vi "Snooze(SubVI).vi"(10 "snooze":dbl, 11 "Time hh::mm":string) -> (3 "Time hh::mm + snooze":string)   [LabVIEW 2023]
doc: "Adds snooze to input time"
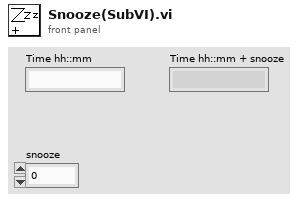
[diagram p1: front panel]
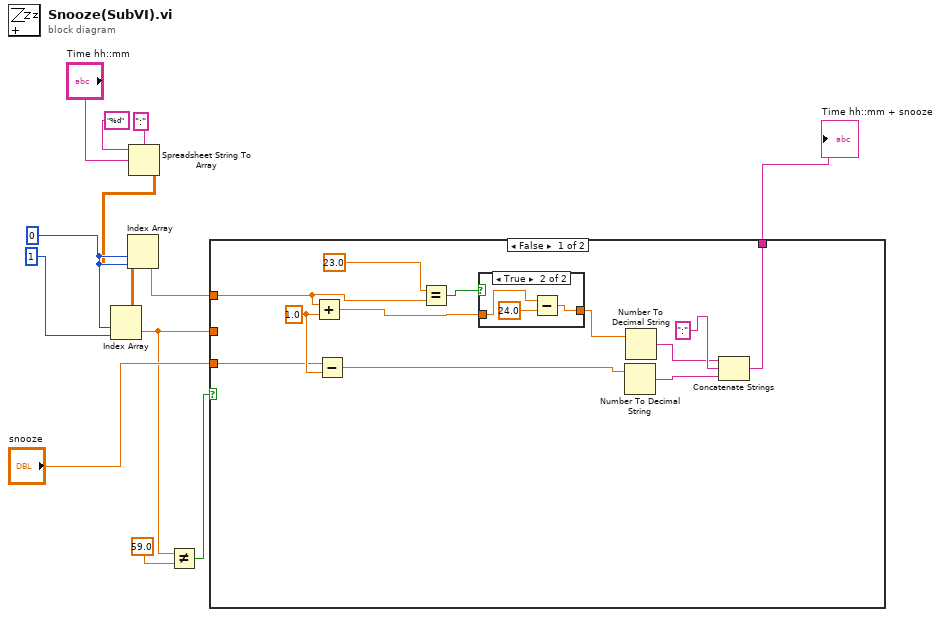
[diagram p0: block diagram]
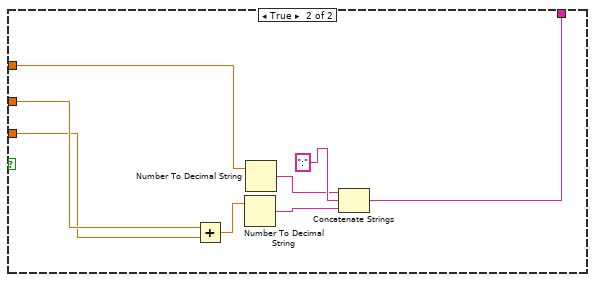
[diagram p3: hidden frame]
diagram:
  w12 = 0 ("index (row)")
  n1 = Spreadsheet String To Array(delimiter (Tab)=":", format string="%d", spreadsheet string="Time hh::mm") -> (array=w8:dbl[][])  [unwired: 1 in]
  n2 = Index Array(array=w8, index (row)=w12, index (col)=1 ("disabled index (col)")) -> (element=w3:dbl)
  n3 = Index Array(array=w8, index (row)=w12, index (col)=w12) -> (element=w10:dbl)
  n4 = Not Equal?(x=w3, y=59.0) -> (x != y?=w1:bool)
  n5 = case shown="False" w1 {
    tunnel: [w21 w36] -> w11
    tunnel: w10 -> [w13 w34]
    tunnel: w3 -> [_ w30]
    tunnel: "snooze" -> [w19 w29]
    frame False {
      w20 = 1.0 ("y")
      n6 = Add(x=w13, y=w20) -> (x+y=w14:dbl)
      n7 = Subtract(x=w19, y=w20) -> (x-y=w18:dbl)
      n8 = Equal?(x=23.0 ("y"), y=w13) -> (x = y?=w17:bool)
      n9 = case shown="True" w17 {
        tunnel: w14 -> [w25 w27]
        tunnel: [w25 w26] -> w16
        frame False {
        }
        frame True {
          n10 = Subtract(x=w27, y=24.0) -> (x-y=w26:dbl)
        }
      }
      n11 = Number To Decimal String(number=w18) -> (decimal integer string=w23:string)  [unwired: 1 in]
      n12 = Number To Decimal String(number=w16) -> (decimal integer string=w22:string)  [unwired: 1 in]
      n13 = Concatenate Strings(w22, ":" ("string"), w23) -> (w21:string)
    }
    frame True {
      n14 = Add(x=w30, y=w29) -> (x+y=w33:dbl)
      n15 = Number To Decimal String(number=w33) -> (decimal integer string=w32:string)  [unwired: 1 in]
      n16 = Number To Decimal String(number=w34) -> (decimal integer string=w31:string)  [unwired: 1 in]
      n17 = Concatenate Strings(w31, ":" ("string"), w32) -> (w36:string)
    }
  }
  "Time hh::mm + snooze" <- w11
